vi "Get Value as Variant.vi"(8 "error in (no error)":errorcluster, 11 "CVT_I32 in":refnum<class "CVT_I32.lvclass">) -> (0 "error out":errorcluster, 2 "data":variant, 3 "CVT_I32 out":refnum<class "CVT_I32.lvclass">)   [LabVIEW 2024, in "Current Value Table.lvlib" / "CVT_I32.lvclass"]
uses:
  CVT_I32.lvclass
  CVT_I32.lvclass/CVT_I32.ctl
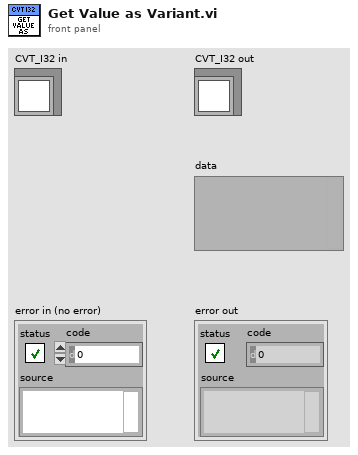
[diagram p1: front panel]
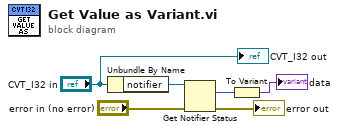
[diagram p0: block diagram]
diagram:
  n1 = Unbundle By Name("CVT_I32 in") -> ("notifier"=w5:refnum<notifier>)
  n2 = Get Notifier Status(notifier=w5, error in (no error)="error in (no error)") -> (current notification=w2:i32, error out=→"error out":errorcluster)  [unwired: 3 out]
  n3 = To Variant(anything=w2) -> (Variant=→"data":variant)
  "CVT_I32 out" <- "CVT_I32 in"
